vi "Tools_String Launch Browser with URL.vi"(4 "error in (no error)":errorcluster, 5 "show dialog (T)":bool=TRUE, 6 "name":string, 7 "url":string) -> (0 "error out":errorcluster)   [LabVIEW 2017]
panel:
  in  "?":refnum<vi>
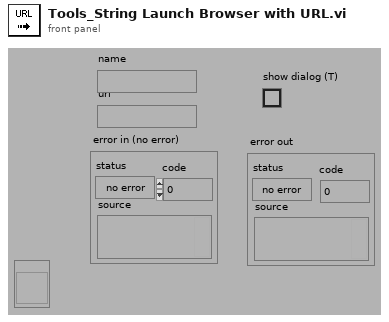
[diagram p1: front panel]
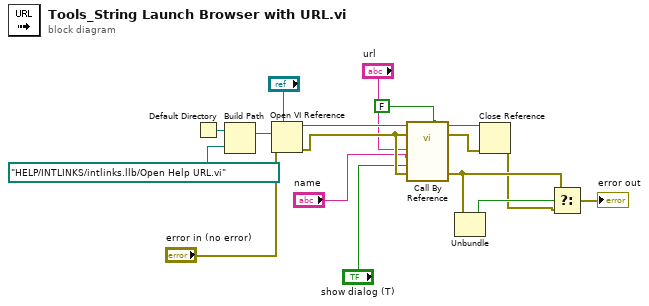
[diagram p0: block diagram]
diagram:
  n1 = Default Directory() -> (w14:path)
  n2 = Build Path(base path=w14, name or relative path=path "HELP/INTLINKS/intlinks.llb/Open Help URL.vi" ("vi path")) -> (appended path=w15:path)
  n3 = Open VI Reference(type specifier VI Refnum (for type only)="?", vi path=w15, error in (no error)="error in (no error)") -> (vi reference=w13:refnum<vi>, error out=w9:errorcluster)  [unwired: 3 out]
  n4 = call-by-ref "?"(reference=w13, error in=w9, "close caller (T)"=FALSE, "error in (no error)"=w9, "show dialog (T)"="show dialog (T)", "name"="name", "url"="url") -> (reference out=w12:refnum<vi>, error out=w11:errorcluster, "error out"=w7:errorcluster)  [unwired: 2 in]
  n5 = Unbundle(w7) -> ("status"=w8:bool)  [unwired: 2 out]
  n6 = Close Reference(reference=w12, error in (no error)=w11) -> (error out=w6:errorcluster)
  n7 = Select(t=w7, s=w8, f=w6) -> (s? t:f=→"error out":errorcluster)
